vi "Configuration.vi"(6 "Return Data":refnum<user-event>, 8 "error in (no error)":errorcluster, 9 "Exit Running Config":refnum<user-event>, 10 "Panel in":refnum<class "Panel.lvclass">, 11 "Numeric Data Type in":refnum<class "Numeric Data Type.lvclass">) -> (0 "error out":errorcluster, 3 "Numeric Data Type out":refnum<class "Numeric Data Type.lvclass">)   [LabVIEW 2018, in "Numeric Data Type.lvclass"]
uses:
  Numeric Data Type.lvclass
  Format Code Type List Enum.ctl
  Date Format.ctl
  Time Format.ctl
  Date Order.ctl
  Year Format.ctl
  Clock Type.ctl
  Padding.ctl
  Precision Type.ctl
  D:/Code/QControls Extended/DataGrid/DataGrid Configuration/Data Type Classes/Generic/Generic Data Type.lvclass
  <vilib>/MGI/Panel Manager/Panel/Panel/Panel.lvclass
  Generic/Generic Data Type.lvclass
  Representation Ring.ctl
  Response to Values Outside of Limits Enum.ctl
  <vilib>/fxp/FXPxcontrol/FXP.xctl
  Generic/Generic Data Type.lvclass/Generic Data Type.ctl
  Numeric Data Type.lvclass/Numeric Data Type.ctl
  Generic/Write Column Header.vi
  Reference Format String.vi
panel:
  in  "Main Tab":T1(tab)
  in  "Default Value (Date/Time)":timestamp
  in  "Default Value (Complex)":cdb=-inf+0.0i caption="Minimum" format="%.4g"
  in  "Default Value":dbl=-inf caption="Minimum" format="%.4g"
  in  "Column Header":string
  in  "FXP":cluster{"Encoding":T2, "Range":T3}(xcontrol)
  in  "Representation":T4
  in  "Use Default Limits":bool
  in  "Limits Mode Tab":enum32{"Numeric", "Timestamp"}(tab)
  in  "Minimum":dbl=-inf format="%.6f"
  in  "Maximum":dbl=inf format="%.6f"
  in  "Minimum Time":timestamp caption="Minimum"
  in  "Maximum Time":timestamp caption="Maximum"
  in  "Increment":dbl format="%.6f"
  in  "Min/Max Warning":string="The value for Minimum  is greater than the value for Maximum.  Adjust the values so that Minumum is less than Maximum." caption="Typedef Message"
  in  "Coerce Minimum":T5 caption="Response to value outside limits"
  in  "Coerce Maximum":T5 caption="Response to value outside limits"
  in  "Coerce Increment":T5 caption="Response to value outside limits"
  in  "Default/Advanced Tab":enum32{"Standard", "Advanced"}(tab)
  in  "Time/Numeric Tab":enum32{"numeric", "time"}(tab)
  in  "Padding":T6 caption="just/pad"
  in  "Use Min Width":bool caption="Use minimum field width"
  in  "Hide Zeroes":bool caption="Hide trailing zeros"
  in  "Exponent":bool caption="Exponent in multiples of 3"
  in  "Precision Type":T7
  in  "Digits":i32=5 min=0
  in  "Min Field Width":i32 caption="Minimum field width"
  in  "Include Seconds":bool caption="Include Seconds?"
  in  "Date Format":T8=enum."System date format" caption="Date Type"
  in  "HMS Digits":i16 caption="Digits" min=0
  in  "Time Format":T9=enum."System time format" caption="Time Type"
  in  "Date Order":T10
  in  "Year Format":T11
  in  "Clock Type":T12
  in  "Type":i32(listbox)
  in  "Revert":bool
  in  "List Type":T13 caption="HLP_Format Code List Type"
  out "Valid":bool=TRUE
  in  "Insert":bool caption="Insert into Format String"
  in  "Format Codes":i32(listbox) caption="Numeric Format Codes"
  in  "Format String":string caption="Format string"
  in  "Editing Mode":enum32{"Default Mode", "Advanced Mode"}(radio)
  # "Numeric Column"
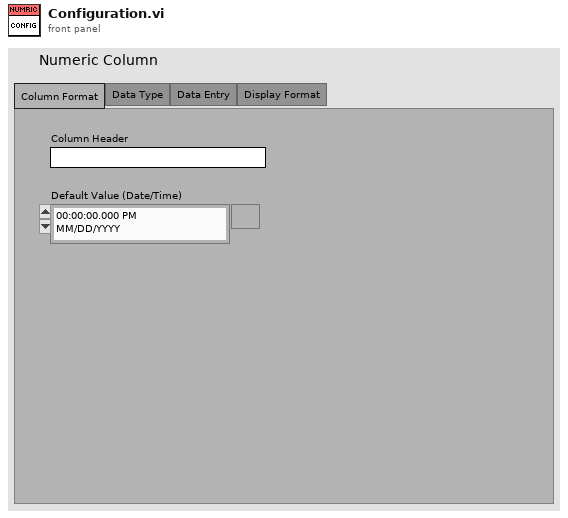
[diagram p1: front panel]
types:
  T1 = enum32{"Column Format", "Data Type", "Data Entry", "Display Format"}
  T2 = typedef "LVFixedPointRepBitsTypeDef.ctl" = cluster{"Signed":bool, "Word Length":u32, "Integer Word Length":i32}
  T3 = typedef "LVFixedPointRepRangeTypeDef.ctl" = cluster{"Range Min":dbl, "Range Max":dbl, "Delta":dbl}
  T4 = typedef "Numeric Data Type.lvclass/Representation Ring.ctl" = u16
  T5 = typedef "Numeric Data Type.lvclass/Response to Values Outside of Limits Enum.ctl" = enum16{"Ignore", "Coerce to nearest", "Coerce up", "Coerce down"}
  T6 = typedef "Numeric Data Type.lvclass/Padding.ctl" = enum16{"Pad with spaces on left", "Pad with spaces on right", "Pad with zeros on left"}
  T7 = typedef "Numeric Data Type.lvclass/Precision Type.ctl" = enum16{"Digits of precision", "Significant digits"}
  T8 = typedef "Numeric Data Type.lvclass/Date Format.ctl" = enum16{"Custom date format", "System date format", "Date unused"}
  T9 = typedef "Numeric Data Type.lvclass/Time Format.ctl" = enum16{"Custom time format", "System time format", "Time unused"}
  T10 = typedef "Numeric Data Type.lvclass/Date Order.ctl" = enum32{"M/D/Y", "D/M/Y", "Y/M/D"}
  T11 = typedef "Numeric Data Type.lvclass/Year Format.ctl" = enum32{"No Year", "2-digit Year", "4-digit Year"}
  T12 = typedef "Numeric Data Type.lvclass/Clock Type.ctl" = enum32{"12-Hour (AM/PM)", "24-Hour"}
  T13 = typedef "Numeric Data Type.lvclass/Format Code Type List Enum.ctl" = enum16{"Numeric format codes", "Relative time format codes", "Absolute time format codes"}
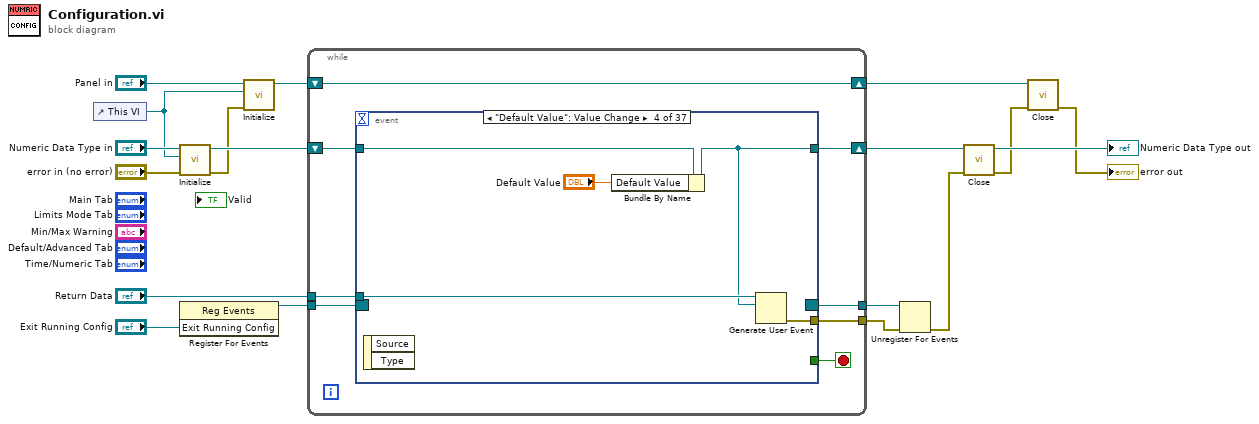
[diagram p0: block diagram]
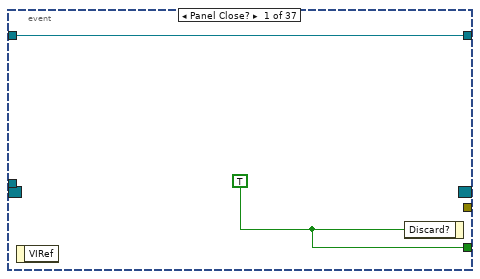
[diagram p2: hidden frame]
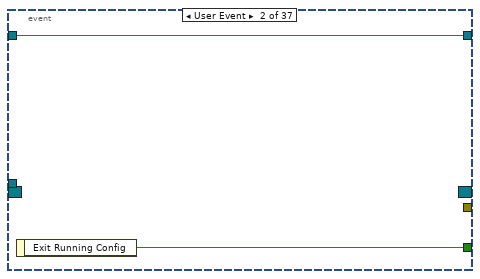
[diagram p3: hidden frame]
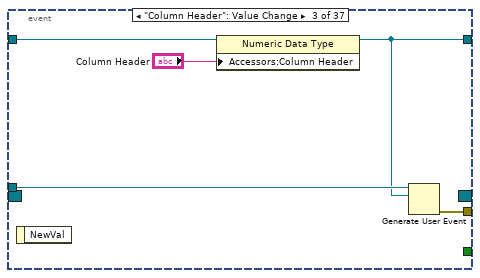
[diagram p4: hidden frame]
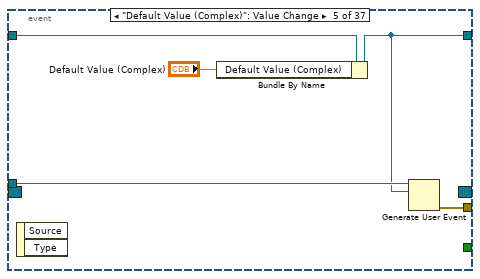
[diagram p5: hidden frame]
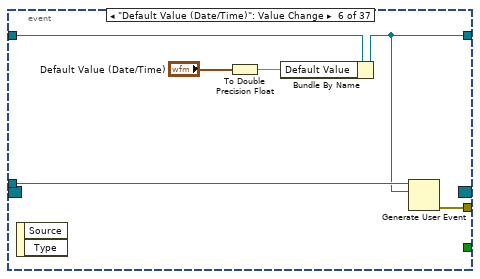
[diagram p6: hidden frame]
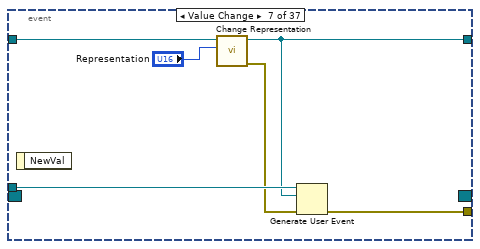
[diagram p7: hidden frame]
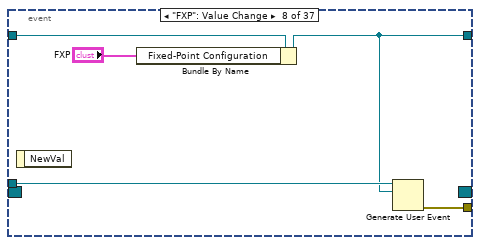
[diagram p8: hidden frame]
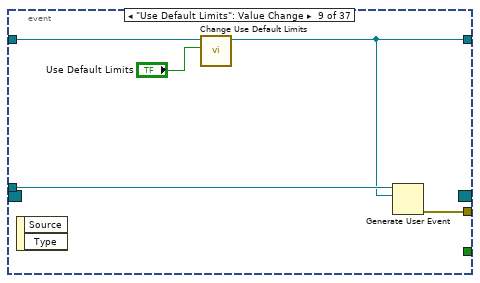
[diagram p9: hidden frame]
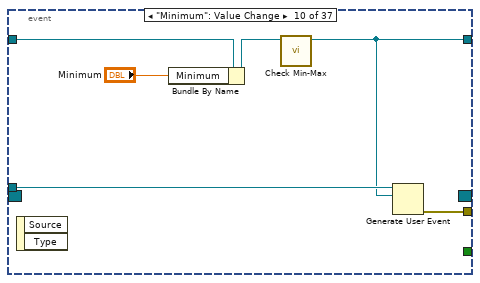
[diagram p10: hidden frame]
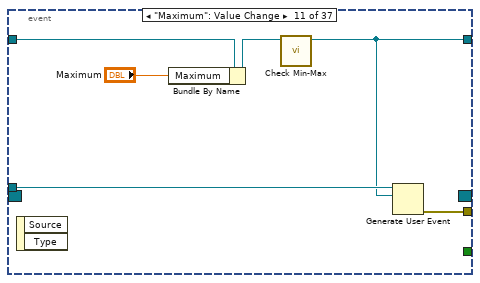
[diagram p11: hidden frame]
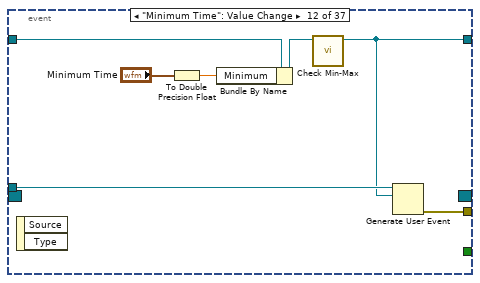
[diagram p12: hidden frame]
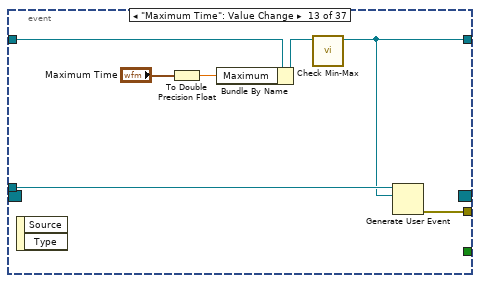
[diagram p13: hidden frame]
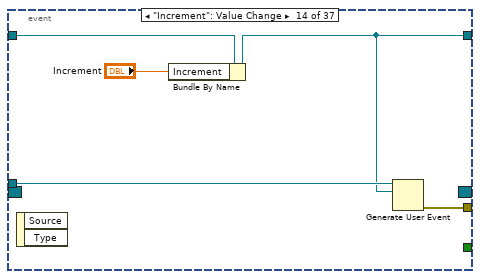
[diagram p14: hidden frame]
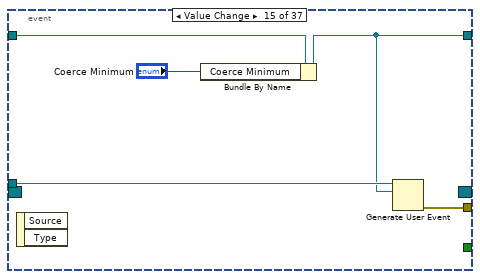
[diagram p15: hidden frame]
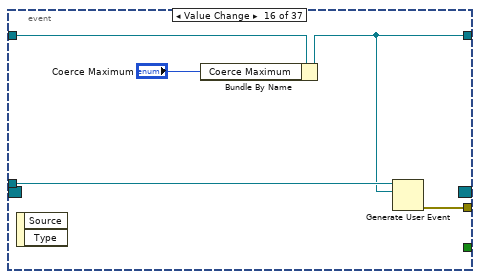
[diagram p16: hidden frame]
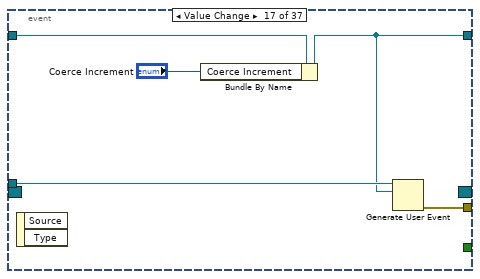
[diagram p17: hidden frame]
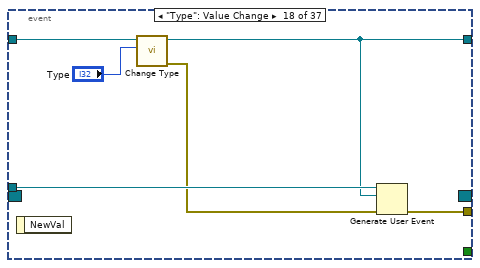
[diagram p18: hidden frame]
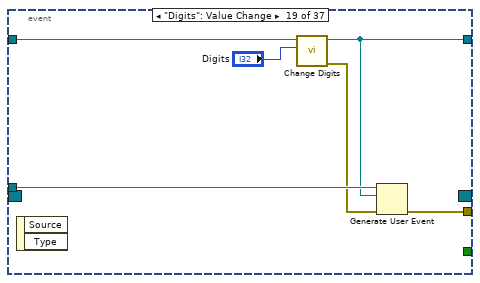
[diagram p19: hidden frame]
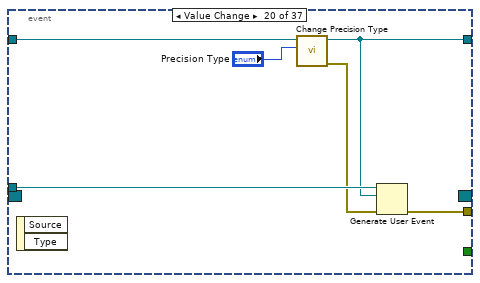
[diagram p20: hidden frame]
diagram:
  n1 = control-ref of="This VI"() -> (w7:refnum<vi>)
  n2 = call <vilib>:"Initialize.vi"("error in (no error)"="error in (no error)", "Main VI"=w7, "Numeric Data Type in"="Numeric Data Type in") -> ("error out"=w5:errorcluster, "Numeric Data Type out"=w13:refnum<class "Numeric Data Type.lvclass">)  [unwired: 7 in]
  n3 = register-events("Exit Running Config") -> (reference out=w17:refnum<event-registration>)  [unwired: 2 in, 1 out]
  n4 = call <vilib>:"Initialize.vi"("error in (no error)"=w5, "VI Refnum"=w7, "Panel In"="Panel in") -> ("Panel Out"=w4:refnum<class "Panel.lvclass">)  [unwired: 6 in, 2 out]
  n5 = while {
    shift-right: [w22] -> w12
    shift-left: w13 -> [w26]
    tunnel: w17 -> [w24]
    tunnel: [w23] -> w16
    tunnel: "Return Data" -> [w21]
    tunnel: [w20] -> w18
    shift-right: [w19] -> w3
    shift-left: w4 -> [w19]
    stop <- w25 stop-if-true
    n6 = event shown="[3] \"Default Value\": Value Change" {
      selector: w24 -> [_ _ _ _ _ _ _ _ _ _ _ _ _ _ _ _ _ _ _ _ _ _ _ _ _ _ _ _ _ _ _ _ _ _ _ _ _]
      dyn-events: [_ _ _ _ _ _ _ _ _ _ _ _ _ _ _ _ _ _ _ _ _ _ _ _ _ _ _ _ _ _ _ _ _ _ _ _ _] -> w23
      timeout: _ -> [_ _ _ _ _ _ _ _ _ _ _ _ _ _ _ _ _ _ _ _ _ _ _ _ _ _ _ _ _ _ _ _ _ _ _ _ _]
      tunnel: w26 -> [w28 w30 w33 w38 w43 w49 w57 w59 w67 w70 w77 w84 w91 w96 w101 w106 w111 w119 w123 w129 w135 w141 w149 w155 w161 w167 w173 w179 w185 w191 w197 w203 w209 w216 w219 w221 w226]
      tunnel: [w28 w30 w32 w37 w42 w48 w55 w58 w64 w68 w75 w82 w89 w94 w99 w105 w110 w114 w122 w128 w134 w140 w148 w154 w160 w166 w172 w178 w184 w190 w196 w202 w208 w216 w217 w222 w225] -> w22
      tunnel: [w27 w29 _ _ _ _ _ _ _ _ _ _ _ _ _ _ _ _ _ _ _ _ _ _ _ _ _ _ _ _ _ _ _ _ _ _ _] -> w25
      tunnel: w21 -> [_ _ w35 w40 w45 w51 w56 w62 w65 w73 w79 w86 w93 w98 w103 w108 w113 w117 w125 w131 w137 w143 w151 w157 w163 w169 w175 w181 w187 w193 w199 w205 w211 _ _ w224 _]
      tunnel: [_ _ w34 w39 w44 w50 w54 w61 w63 w72 w78 w85 w92 w97 w102 w107 w112 w115 w124 w130 w136 w142 w150 w156 w162 w168 w174 w180 w186 w192 w198 w204 w210 w212 _ w223 _] -> w20
      event Panel Close? {
        w27 = TRUE
        n7 = event-data() -> ()  [unwired: 1 in, 1 out]
        n8 = event-data("Discard?"=w27) -> ()  [unwired: 1 in, 1 out]
      }
      event User Event {
        n9 = event-data() -> ("Exit Running Config"=w29:bool)  [unwired: 1 in]
      }
      event "Column Header": Value Change {
        n10 = event-data() -> ()  [unwired: 1 in, 1 out]
        n11 = property class="Numeric Data Type"(reference=w33, "Accessors:Column Header"="Column Header") -> (reference out=w32:refnum<class "Numeric Data Type.lvclass">)  [unwired: 1 in, 1 out]
        n12 = Generate User Event(user event=w35, event data cluster=w32) -> (error out=w34:errorcluster)  [unwired: 2 in, 1 out]
      }
      event "Default Value": Value Change {
        n13 = event-data() -> ()  [unwired: 1 in, 2 out]
        n14 = Bundle By Name(cluster=w38, "Default Value"="Default Value") -> (w37:refnum<class "Numeric Data Type.lvclass">)
        n15 = Generate User Event(user event=w40, event data cluster=w37) -> (error out=w39:errorcluster)  [unwired: 2 in, 1 out]
      }
      event "Default Value (Complex)": Value Change {
        n16 = event-data() -> ()  [unwired: 1 in, 2 out]
        n17 = Bundle By Name(cluster=w43, "Default Value (Complex)"="Default Value (Complex)") -> (w42:refnum<class "Numeric Data Type.lvclass">)
        n18 = Generate User Event(user event=w45, event data cluster=w42) -> (error out=w44:errorcluster)  [unwired: 2 in, 1 out]
      }
      event "Default Value (Date/Time)": Value Change {
        n19 = event-data() -> ()  [unwired: 1 in, 2 out]
        n20 = To Double Precision Float(number="Default Value (Date/Time)") -> (double precision float=w47:dbl)
        n21 = Bundle By Name(cluster=w49, "Default Value"=w47) -> (w48:refnum<class "Numeric Data Type.lvclass">)
        n22 = Generate User Event(user event=w51, event data cluster=w48) -> (error out=w50:errorcluster)  [unwired: 2 in, 1 out]
      }
      event Value Change {
        n23 = event-data() -> ()  [unwired: 1 in, 1 out]
        n24 = call "Change Representation.vi"("Representation"="Representation", "Numeric Data Type in"=w57) -> ("error out"=w52:errorcluster, "Numeric Data Type out"=w55:refnum<class "Numeric Data Type.lvclass">)  [unwired: 8 in]
        n25 = Generate User Event(user event=w56, event data cluster=w55, error in=w52) -> (error out=w54:errorcluster)  [unwired: 1 in, 1 out]
      }
      event "FXP": Value Change {
        n26 = event-data() -> ()  [unwired: 1 in, 1 out]
        n27 = Bundle By Name(cluster=w59, "Fixed-Point Configuration"="FXP") -> (w58:refnum<class "Numeric Data Type.lvclass">)
        n28 = Generate User Event(user event=w62, event data cluster=w58) -> (error out=w61:errorcluster)  [unwired: 2 in, 1 out]
      }
      event "Use Default Limits": Value Change {
        n29 = event-data() -> ()  [unwired: 1 in, 2 out]
        n30 = call "Change Use Default Limits.vi"("Use Default Limits"="Use Default Limits", "Numeric Data Type in"=w67) -> ("Numeric Data Type out"=w64:refnum<class "Numeric Data Type.lvclass">)  [unwired: 8 in, 1 out]
        n31 = Generate User Event(user event=w65, event data cluster=w64) -> (error out=w63:errorcluster)  [unwired: 2 in, 1 out]
      }
      event "Minimum": Value Change {
        n32 = event-data() -> ()  [unwired: 1 in, 2 out]
        n33 = Bundle By Name(cluster=w70, "Minimum"="Minimum") -> (w69:refnum<class "Numeric Data Type.lvclass">)
        n34 = call "Check Min-Max.vi"("Numeric Data Type in"=w69) -> ("Numeric Data Type (dup)"=w68:refnum<class "Numeric Data Type.lvclass">)  [unwired: 9 in, 1 out]
        n35 = Generate User Event(user event=w73, event data cluster=w68) -> (error out=w72:errorcluster)  [unwired: 2 in, 1 out]
      }
      event "Maximum": Value Change {
        n36 = event-data() -> ()  [unwired: 1 in, 2 out]
        n37 = Bundle By Name(cluster=w77, "Maximum"="Maximum") -> (w76:refnum<class "Numeric Data Type.lvclass">)
        n38 = call "Check Min-Max.vi"("Numeric Data Type in"=w76) -> ("Numeric Data Type (dup)"=w75:refnum<class "Numeric Data Type.lvclass">)  [unwired: 9 in, 1 out]
        n39 = Generate User Event(user event=w79, event data cluster=w75) -> (error out=w78:errorcluster)  [unwired: 2 in, 1 out]
      }
      event "Minimum Time": Value Change {
        n40 = event-data() -> ()  [unwired: 1 in, 2 out]
        n41 = To Double Precision Float(number="Minimum Time") -> (double precision float=w81:dbl)
        n42 = Bundle By Name(cluster=w84, "Minimum"=w81) -> (w83:refnum<class "Numeric Data Type.lvclass">)
        n43 = call "Check Min-Max.vi"("Numeric Data Type in"=w83) -> ("Numeric Data Type (dup)"=w82:refnum<class "Numeric Data Type.lvclass">)  [unwired: 9 in, 1 out]
        n44 = Generate User Event(user event=w86, event data cluster=w82) -> (error out=w85:errorcluster)  [unwired: 2 in, 1 out]
      }
      event "Maximum Time": Value Change {
        n45 = event-data() -> ()  [unwired: 1 in, 2 out]
        n46 = To Double Precision Float(number="Maximum Time") -> (double precision float=w88:dbl)
        n47 = Bundle By Name(cluster=w91, "Maximum"=w88) -> (w90:refnum<class "Numeric Data Type.lvclass">)
        n48 = call "Check Min-Max.vi"("Numeric Data Type in"=w90) -> ("Numeric Data Type (dup)"=w89:refnum<class "Numeric Data Type.lvclass">)  [unwired: 9 in, 1 out]
        n49 = Generate User Event(user event=w93, event data cluster=w89) -> (error out=w92:errorcluster)  [unwired: 2 in, 1 out]
      }
      event "Increment": Value Change {
        n50 = event-data() -> ()  [unwired: 1 in, 2 out]
        n51 = Bundle By Name(cluster=w96, "Increment"="Increment") -> (w94:refnum<class "Numeric Data Type.lvclass">)
        n52 = Generate User Event(user event=w98, event data cluster=w94) -> (error out=w97:errorcluster)  [unwired: 2 in, 1 out]
      }
      event Value Change {
        n53 = event-data() -> ()  [unwired: 1 in, 2 out]
        n54 = Bundle By Name(cluster=w101, "Coerce Minimum"="Coerce Minimum") -> (w99:refnum<class "Numeric Data Type.lvclass">)
        n55 = Generate User Event(user event=w103, event data cluster=w99) -> (error out=w102:errorcluster)  [unwired: 2 in, 1 out]
      }
      event Value Change {
        n56 = event-data() -> ()  [unwired: 1 in, 2 out]
        n57 = Bundle By Name(cluster=w106, "Coerce Maximum"="Coerce Maximum") -> (w105:refnum<class "Numeric Data Type.lvclass">)
        n58 = Generate User Event(user event=w108, event data cluster=w105) -> (error out=w107:errorcluster)  [unwired: 2 in, 1 out]
      }
      event Value Change {
        n59 = event-data() -> ()  [unwired: 1 in, 2 out]
        n60 = Bundle By Name(cluster=w111, "Coerce Increment"="Coerce Increment") -> (w110:refnum<class "Numeric Data Type.lvclass">)
        n61 = Generate User Event(user event=w113, event data cluster=w110) -> (error out=w112:errorcluster)  [unwired: 2 in, 1 out]
      }
      event "Type": Value Change {
        n62 = event-data() -> ()  [unwired: 1 in, 1 out]
        n63 = call "Change Type.vi"("Type"="Type", "Numeric Data Type in"=w119) -> ("error out"=w116:errorcluster, "Numeric Data Type out"=w114:refnum<class "Numeric Data Type.lvclass">)  [unwired: 8 in]
        n64 = Generate User Event(user event=w117, event data cluster=w114, error in=w116) -> (error out=w115:errorcluster)  [unwired: 1 in, 1 out]
      }
      event "Digits": Value Change {
        n65 = event-data() -> ()  [unwired: 1 in, 2 out]
        n66 = call "Change Digits.vi"("Digits"="Digits", "Numeric Data Type in"=w123) -> ("error out"=w121:errorcluster, "Numeric Data Type out"=w122:refnum<class "Numeric Data Type.lvclass">)  [unwired: 8 in]
        n67 = Generate User Event(user event=w125, event data cluster=w122, error in=w121) -> (error out=w124:errorcluster)  [unwired: 1 in, 1 out]
      }
      event Value Change {
        n68 = event-data() -> ()  [unwired: 1 in, 2 out]
        n69 = call "Change Precision Type.vi"("Precision Type"="Precision Type", "Numeric Data Type in"=w129) -> ("error out"=w127:errorcluster, "Numeric Data Type out"=w128:refnum<class "Numeric Data Type.lvclass">)  [unwired: 8 in]
        n70 = Generate User Event(user event=w131, event data cluster=w128, error in=w127) -> (error out=w130:errorcluster)  [unwired: 1 in, 1 out]
      }
      event "Hide Zeroes": Value Change {
        n71 = event-data() -> ()  [unwired: 1 in, 2 out]
        n72 = call "Change Hide Trailing Zeros.vi"("Hide trailing zeros"="Hide Zeroes", "Numeric Data Type in"=w135) -> ("error out"=w133:errorcluster, "Numeric Data Type out"=w134:refnum<class "Numeric Data Type.lvclass">)  [unwired: 8 in]
        n73 = Generate User Event(user event=w137, event data cluster=w134, error in=w133) -> (error out=w136:errorcluster)  [unwired: 1 in, 1 out]
      }
      event "Exponent": Value Change {
        n74 = event-data() -> ()  [unwired: 1 in, 2 out]
        n75 = call "Change Exponent.vi"("Exponent"="Exponent", "Numeric Data Type in"=w141) -> ("error out"=w138:errorcluster, "Numeric Data Type out"=w140:refnum<class "Numeric Data Type.lvclass">)  [unwired: 8 in]
        n76 = Generate User Event(user event=w143, event data cluster=w140, error in=w138) -> (error out=w142:errorcluster)  [unwired: 1 in, 1 out]
      }
      event "Use Min Width": Value Change {
        n77 = event-data() -> ()  [unwired: 1 in, 2 out]
        n78 = Boolean To (0,1)(Boolean="Use Min Width") -> (0, 1=w146:i16)
        n79 = To Long Integer(number=w146) -> (32bit integer=w144:i32)
        n80 = call "Change Minimum Field Width.vi"("Minimum Field Width"=w144, "Numeric Data Type in"=w149) -> ("error out"=w147:errorcluster, "Numeric Data Type out"=w148:refnum<class "Numeric Data Type.lvclass">)  [unwired: 8 in]
        n81 = Generate User Event(user event=w151, event data cluster=w148, error in=w147) -> (error out=w150:errorcluster)  [unwired: 1 in, 1 out]
      }
      event "Min Field Width": Value Change {
        n82 = event-data() -> ()  [unwired: 1 in, 2 out]
        n83 = call "Change Minimum Field Width.vi"("Minimum Field Width"="Min Field Width", "Numeric Data Type in"=w155) -> ("error out"=w153:errorcluster, "Numeric Data Type out"=w154:refnum<class "Numeric Data Type.lvclass">)  [unwired: 8 in]
        n84 = Generate User Event(user event=w157, event data cluster=w154, error in=w153) -> (error out=w156:errorcluster)  [unwired: 1 in, 1 out]
      }
      event Value Change {
        n85 = event-data() -> ()  [unwired: 1 in, 2 out]
        n86 = call "Change Padding.vi"("Padding"="Padding", "Numeric Data Type in"=w161) -> ("error out"=w159:errorcluster, "Numeric Data Type out"=w160:refnum<class "Numeric Data Type.lvclass">)  [unwired: 8 in]
        n87 = Generate User Event(user event=w163, event data cluster=w160, error in=w159) -> (error out=w162:errorcluster)  [unwired: 1 in, 1 out]
      }
      event Value Change {
        n88 = event-data() -> ()  [unwired: 1 in, 2 out]
        n89 = call "Change Time Format.vi"("Time Format"="Time Format", "Numeric Data Type in"=w167) -> ("error out"=w165:errorcluster, "Numeric Data Type out"=w166:refnum<class "Numeric Data Type.lvclass">)  [unwired: 8 in]
        n90 = Generate User Event(user event=w169, event data cluster=w166, error in=w165) -> (error out=w168:errorcluster)  [unwired: 1 in, 1 out]
      }
      event Value Change {
        n91 = event-data() -> ()  [unwired: 1 in, 2 out]
        n92 = call "Change Clock Type.vi"("Clock Type"="Clock Type", "Numeric Data Type in"=w173) -> ("error out"=w171:errorcluster, "Numeric Data Type out"=w172:refnum<class "Numeric Data Type.lvclass">)  [unwired: 8 in]
        n93 = Generate User Event(user event=w175, event data cluster=w172, error in=w171) -> (error out=w174:errorcluster)  [unwired: 1 in, 1 out]
      }
      event "Include Seconds": Value Change {
        n94 = event-data() -> ()  [unwired: 1 in, 2 out]
        n95 = call "Change Include Seconds.vi"("Include Seconds?"="Include Seconds", "Numeric Data Type in"=w179) -> ("error out"=w177:errorcluster, "Numeric Data Type out"=w178:refnum<class "Numeric Data Type.lvclass">)  [unwired: 8 in]
        n96 = Generate User Event(user event=w181, event data cluster=w178, error in=w177) -> (error out=w180:errorcluster)  [unwired: 1 in, 1 out]
      }
      event "HMS Digits": Value Change {
        n97 = event-data() -> ()  [unwired: 1 in, 2 out]
        n98 = call "Change HMS Digits.vi"("HMS Digits"="HMS Digits", "Numeric Data Type in"=w185) -> ("error out"=w183:errorcluster, "Numeric Data Type out"=w184:refnum<class "Numeric Data Type.lvclass">)  [unwired: 8 in]
        n99 = Generate User Event(user event=w187, event data cluster=w184, error in=w183) -> (error out=w186:errorcluster)  [unwired: 1 in, 1 out]
      }
      event Value Change {
        n100 = event-data() -> ()  [unwired: 1 in, 2 out]
        n101 = call "Change Date Format.vi"("Time Format"="Date Format", "Numeric Data Type in"=w191) -> ("error out"=w189:errorcluster, "Numeric Data Type out"=w190:refnum<class "Numeric Data Type.lvclass">)  [unwired: 8 in]
        n102 = Generate User Event(user event=w193, event data cluster=w190, error in=w189) -> (error out=w192:errorcluster)  [unwired: 1 in, 1 out]
      }
      event Value Change {
        n103 = event-data() -> ()  [unwired: 1 in, 2 out]
        n104 = call "Change Date Order.vi"("Date Order"="Date Order", "Numeric Data Type in"=w197) -> ("error out"=w195:errorcluster, "Numeric Data Type out"=w196:refnum<class "Numeric Data Type.lvclass">)  [unwired: 8 in]
        n105 = Generate User Event(user event=w199, event data cluster=w196, error in=w195) -> (error out=w198:errorcluster)  [unwired: 1 in, 1 out]
      }
      event Value Change {
        n106 = event-data() -> ()  [unwired: 1 in, 2 out]
        n107 = call "Change Year Format.vi"("Year Format"="Year Format", "Numeric Data Type in"=w203) -> ("error out"=w201:errorcluster, "Numeric Data Type out"=w202:refnum<class "Numeric Data Type.lvclass">)  [unwired: 8 in]
        n108 = Generate User Event(user event=w205, event data cluster=w202, error in=w201) -> (error out=w204:errorcluster)  [unwired: 1 in, 1 out]
      }
      event "Format String": Value Change {
        n109 = event-data() -> ()  [unwired: 1 in, 2 out]
        n110 = call "Change Format String.vi"("Format String"="Format String", "Numeric Data Type in"=w209) -> ("error out"=w207:errorcluster, "Numeric Data Type out"=w208:refnum<class "Numeric Data Type.lvclass">)  [unwired: 8 in]
        n111 = Generate User Event(user event=w211, event data cluster=w208, error in=w207) -> (error out=w210:errorcluster)  [unwired: 1 in, 1 out]
      }
      event "Revert": Value Change {
        n112 = event-data() -> ()  [unwired: 1 in, 2 out]
        n113 = Unbundle By Name(w216) -> ("Format String"=w213:string)
        n114 = call-poly "Reference.vi"() -> ("error out"=w214:errorcluster, "Format String"=w215:refnum<vi>)  [unwired: 10 in]
        n115 = property class="Str"(reference=w215, error in=w214, "Val(Sgnl)"=w213) -> (error out=w212:errorcluster)  [unwired: 1 out]
      }
      event Value Change {
        n116 = event-data() -> ()  [unwired: 1 in, 2 out]
        n117 = call "Change List Type.vi"("List type"="List Type", "Numeric Data Type in"=w219) -> ("Numeric Data Type out"=w217:refnum<class "Numeric Data Type.lvclass">)  [unwired: 8 in, 1 out]
      }
      event "Format Codes": Double Click; "Insert": Value Change {
        n118 = event-data() -> ()  [unwired: 1 in, 2 out]
        n119 = call "Insert Format Code.vi"("Numeric Data Type in"=w221) -> ("error out"=w220:errorcluster, "Numeric Data Type (dup)"=w222:refnum<class "Numeric Data Type.lvclass">)  [unwired: 9 in]
        n120 = Generate User Event(user event=w224, event data cluster=w222, error in=w220) -> (error out=w223:errorcluster)  [unwired: 1 in, 1 out]
      }
      event "Editing Mode": Value Change {
        n121 = event-data() -> ()  [unwired: 1 in, 2 out]
        n122 = call "Change Mode.vi"("Editing Mode"="Editing Mode", "Numeric Data Type in"=w226) -> ("Numeric Data Type out"=w225:refnum<class "Numeric Data Type.lvclass">)  [unwired: 8 in, 1 out]
      }
    }
  }
  n123 = Unregister For Events(event registration refnum=w16, error in=w18) -> (error out=w10:errorcluster)
  n124 = call "Close.vi"("error in (no error)"=w10, "Numeric Data Type in"=w12) -> ("error out"=w2:errorcluster, "Numeric Data Type out"=→"Numeric Data Type out":refnum<class "Numeric Data Type.lvclass">)  [unwired: 8 in]
  n125 = call-dynamic "Close.vi"("Error In"=w2, "Panel In"=w3) -> ("Error Out"=→"error out":errorcluster)  [unwired: 9 in]
